vi "Fix Old Dates in Data File.vi"() -> ()   [LabVIEW 2021]
uses:
  WPC Player and Financial Stats.ctl
panel:
  out "Updated Stats":T1[][](array[typedef]) {"Date Updated" format="%<%m/%d/%Y>T"}
  out "Original Stats":T1[][](array[typedef]) {"Date Updated" format="%<%m/%d/%Y>T"}
  in  "file path (use dialog)":path=path "C:/Users/manma/Google Drive/WPC Stat Scrape/Data/WPC Stats.bin"
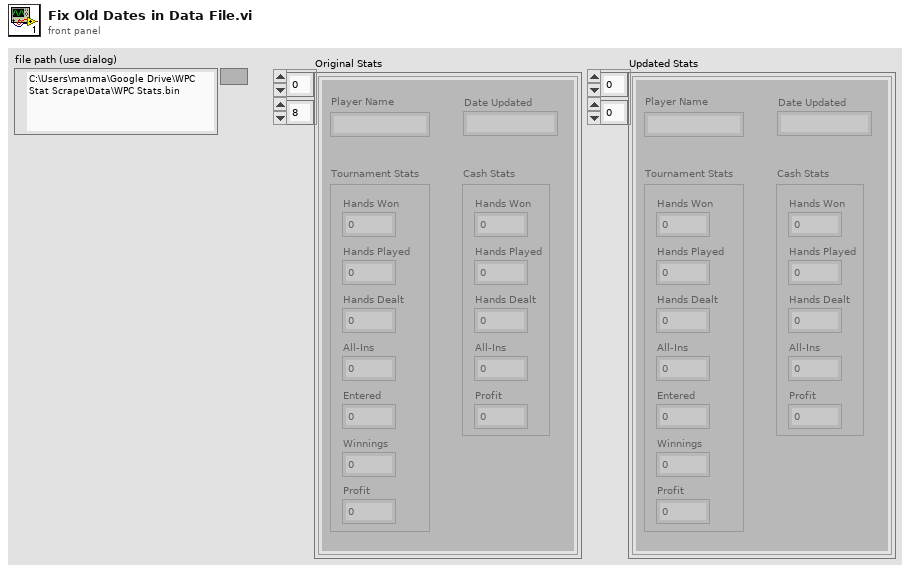
[diagram p1: front panel]
types:
  T1 = typedef "WPC Player and Financial Stats.ctl" = cluster{"Player Name":string, "Date Updated":timestamp, "Tournament Stats":cluster{"Hands Won":i32, "Hands Played":i32, "Hands Dealt":i32, "All-Ins":i32, "Entered":i32, "Winnings":dbl, "Profit":dbl}, "Cash Stats":cluster{"Hands Won":i32, "Hands Played":i32, "Hands Dealt":i32, "All-Ins":i32, "Profit":dbl}}
  T2 = enum16{"open", "replace", "create", "open or create", "replace or create", "replace or create with confirmation"}
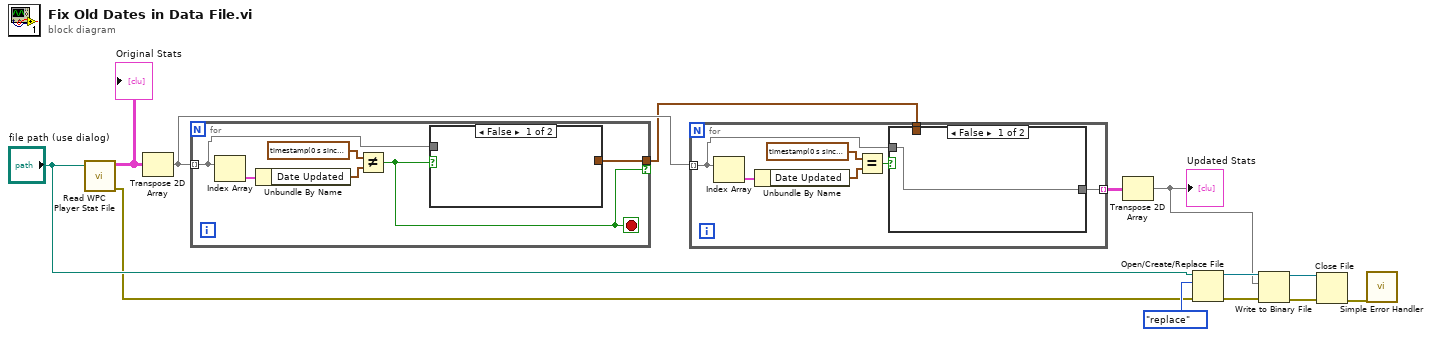
[diagram p0: block diagram]
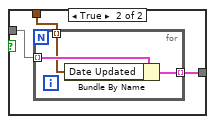
[diagram p2: hidden frame]
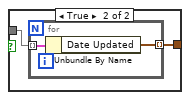
[diagram p3: hidden frame]
diagram:
  n1 = call "Read WPC Player Stat File.vi"("file path (use dialog)"="file path (use dialog)") -> ("error out"=w3:errorcluster, "Full WPC Stats"=w12:T1[][])  [unwired: 8 in, 1 out]
  "Original Stats" <- w12
  n2 = Transpose 2D Array(2D array=w12) -> (transposed array=w11:T1[][])
  n3 = for {
    tunnel: w11 -> [w16] mode=indexing
    tunnel: [w15] -> w10 if=w14
    stop <- w14 stop-if-true
    n4 = Index Array(array=w16) -> (element=w19:T1)  [unwired: 1 in]
    n5 = Unbundle By Name(w19) -> ("Date Updated"=w17:timestamp)
    n6 = Not Equal?(x=timestamp(0 s since 1904-01-01) ("Date Updated"), y=w17) -> (x != y?=w14:bool)
    n7 = case shown="False" w14 {
      tunnel: w16 -> [_ w21]
      tunnel: [_ w20] -> w15
      frame False {
      }
      frame True {
        n8 = for {
          tunnel: w21 -> [w23] mode=indexing
          tunnel: [w22] -> w20 mode=indexing
          n9 = Unbundle By Name(w23) -> ("Date Updated"=w22:timestamp)
        }
      }
    }
  }
  n10 = for {
    tunnel: w11 -> [w27] mode=indexing
    tunnel: w10 -> [w24]
    tunnel: [w25] -> w9 mode=indexing
    n11 = Index Array(array=w27) -> (element=w30:T1)  [unwired: 1 in]
    n12 = Unbundle By Name(w30) -> ("Date Updated"=w28:timestamp)
    n13 = Equal?(x=timestamp(0 s since 1904-01-01) ("Date Updated"), y=w28) -> (x = y?=w26:bool)
    n14 = case shown="False" w26 {
      tunnel: w27 -> [w31 w34]
      tunnel: [w31 w33] -> w25
      tunnel: w24 -> [_ w32]
      frame False {
      }
      frame True {
        n15 = for {
          tunnel: w34 -> [w37] mode=indexing
          tunnel: [w36] -> w33 mode=indexing
          tunnel: w32 -> [w35] mode=indexing
          n16 = Bundle By Name(cluster=w37, "Date Updated"=w35) -> (w36:T1)
        }
      }
    }
  }
  n17 = Transpose 2D Array(2D array=w9) -> (transposed array=w2:T1[][])
  "Updated Stats" <- w2
  n18 = Open/Create/Replace File(file path (use dialog)="file path (use dialog)", error in=w3, operation (0:open)=T2."replace") -> (refnum out=w6:refnum<file>, error out=w7:errorcluster)  [unwired: 3 in, 1 out]
  n19 = Write to Binary File(file (use dialog)=w6, data=w2, error in=w7) -> (refnum out=w5:refnum<file>, error out=w4:errorcluster)  [unwired: 3 in, 1 out]
  n20 = Close File(refnum=w5, error in=w4) -> (error out=w1:errorcluster)  [unwired: 1 out]
  n21 = call <vilib>:"Simple Error Handler.vi"("error in (no error)"=w1) -> ()  [unwired: 4 in, 5 out]
